vi "DB String Array.vi"() -> (3 "DB string array":i8[][](array[numeric]))   [LabVIEW 2017, in "Database.lvlib"]
uses:
  Database.lvlib
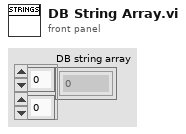
[diagram p1: front panel]
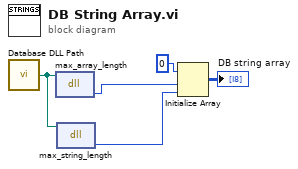
[diagram p0: block diagram]
diagram:
  n1 = call "Database DLL Path.vi"() -> ("DLL Path"=w4:path)  [unwired: 5 in]
  n2 = dll-call lib="?" fn="max_array_length"(path in=w4) -> ("return type"=w3:i32)  [unwired: 2 in, 2 out]
  n3 = dll-call lib="?" fn="max_string_length"(path in=w4) -> ("return type"=w2:i32)  [unwired: 2 in, 2 out]
  n4 = Initialize Array(i8 0 ("element"), w3, w2) -> (→"DB string array":i8[][])
